vi "DG535 Check Status.vi"(8 "error in":errorcluster, 11 "VISA resource name":refnum<visa-resource-name>) -> (0 "error out":errorcluster, 1 "offset past number":i32, 2 "Status byte":i32 format="%b", 3 "VISA resource name out":refnum<visa-resource-name>)   [LabVIEW 2020]
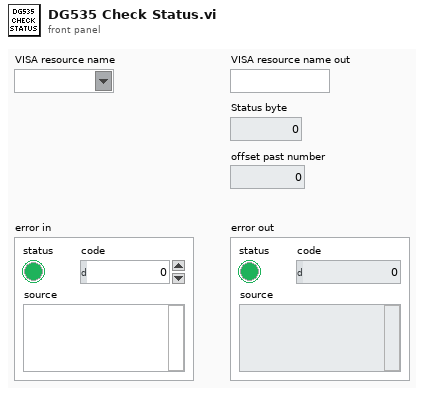
[diagram p1: front panel]
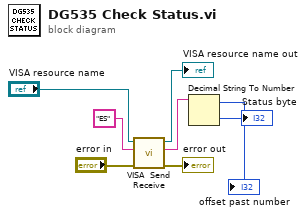
[diagram p0: block diagram]
diagram:
  n1 = call "VISA  Send Receive.vi"("error in (no error)"="error in", "data string in"="ES" ("format string"), "VISA Resource Name"="VISA resource name") -> ("error out"=→"error out":errorcluster, "data string out"=w3:string, "VISA Resource Name Out"=→"VISA resource name out":refnum<visa-resource-name>)  [unwired: 6 in]
  n2 = Decimal String To Number(string=w3) -> (offset past number=→"offset past number":i32, number=→"Status byte":i32)  [unwired: 2 in]
